vi "Control Intake Reverse.vi"(11 "Avoid Race Condition":bool) -> ()   [LabVIEW 2020]
uses:
  Framework/Robot Global Data.vi
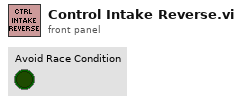
[diagram p1: front panel]
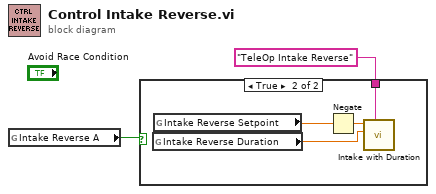
[diagram p0: block diagram]
diagram:
  n1 = global read "Robot Global Data.vi" "Intake Reverse A"() -> (w2:bool)
  n2 = case shown="True" w2 {
    tunnel: "TeleOp Intake Reverse" ("Description") -> [_ w6]
    frame False {
    }
    frame True {
      n3 = global read "Robot Global Data.vi" "Intake Reverse Duration"() -> (w3:dbl)
      n4 = global read "Robot Global Data.vi" "Intake Reverse Setpoint"() -> (w4:dbl)
      n5 = Negate(x=w4) -> (-x=w5:dbl)
      n6 = call "Intake with Duration.vi"("Description"=w6, "Duration (s)"=w3, "Setpoint"=w5) -> ()  [unwired: 8 in, 1 out]
    }
  }
